vi "SiPM_Tests_Global_Var.vi"() -> ()   [LabVIEW 2019]
uses:
  <vilib>/Analysis/6fits.llb/Curve Fitting Criteria.ctl
  <vilib>/Analysis/NI_AALPro.lvlib
panel:
  in  "Dead Time":u16=100
  in  "Trigger Source":T1(ring)
  out "Channel Name":string
  out "Group_Name":string
  in  "Nb of Laser Pulses":u8
  in  "Trig Delay":u8
  in  "Trig Length":u8
  out "FIFO_pkt_size":u16
  in  "Measurement":string
  in  "Spectrum Only":bool
  in  "System Type":bool=TRUE
  in  "Edge Det\nDis":bool
  in  "Integr_dur":sgl(slide) min=0 max=12.75 step=0.05 scale=0.0..12.0 scale format="%#.2f"
  in  "Trigger thr":sgl(slide) min=0 max=3.3 step=0.001 scale=0.0..3.3
  out "DAQ-Error":errorcluster
  out "DAQ-VISA":refnum<visa-resource-name>
  in  "Wvfm Stop":i32=2 caption="Wvfm Stop (ns)"
  in  "Wvfm Start":i32=2 caption="Wvfm Start (ns)"
  in  "NbSamples":u16 caption="Nb of Samples to Analyze"
  in  "width":i32
  in  "threshold":dbl
  in  "method":T2=1 items=["Least Square", "Least Absolute Residual", "Bisquare"]
  in  "Init_std_dev":dbl=1.0
  in  "Offset":i32
  in  "Nb of Samples to Display":i32=50
  in  "TDMS file array":refnum<k34>[](array[refnum])
  in  "Waveform Nb":u16
  in  "Attenuation":dbl
  in  "Delay (ns)":dbl
  in  "Save Results?":bool
  out "Default?":bool
  out "App Dir":path
  in  "Directory":path=path "C:/Users/johnk/Desktop/ESA_Scintillator_Data"
  in  "File Name":string="1"
  out "Y-Home":dbl
  out "X-Home":dbl
  in  "Arduino Error":errorcluster
  in  "Arduino VISA":refnum<visa-resource-name>
  in  "Hist Min":dbl format="%0.2f"
  in  "Hist Max":dbl format="%0.2f"
  out "Pulser VISA":refnum<visa-resource-name>
  out "Pulser Error":errorcluster
  out "PwrSupply VISA":refnum<visa-resource-name>
  out "PwrSupply Error":errorcluster
  out "Scope Error":errorcluster
  out "Scope VISA":refnum<visa-resource-name>
  in  "Session Log ref":refnum<vi>
  # "PIFN System Config"
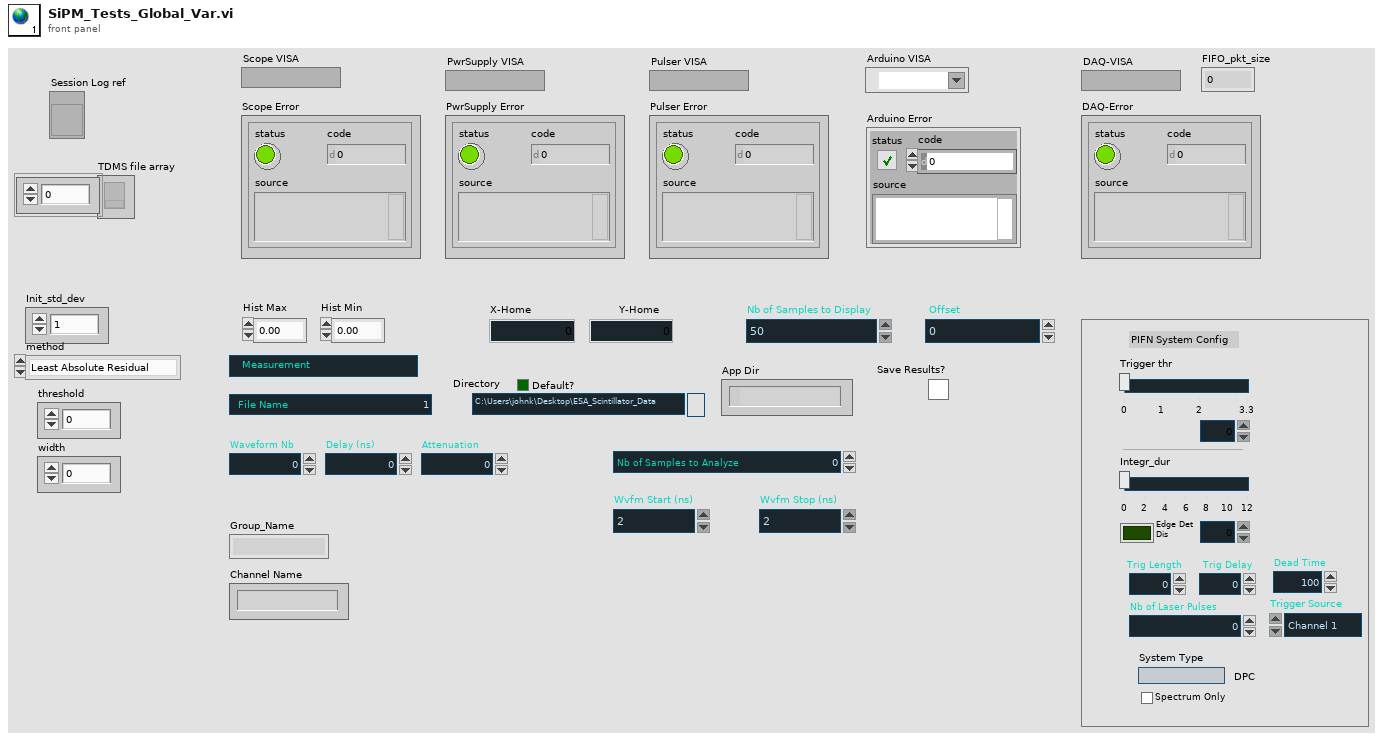
[diagram p1: front panel]
types:
  T1 = enum16{"Channel 1", "Channel 2", "Channel 3", "Channel 4", "Channel 5", "Channel 6"}
  T2 = typedef "NI_AALPro.lvlib/Curve Fitting Criteria.ctl" = u16
diagram:
